vi "Set US Genomics.vi"(8 "error in (no error)":errorcluster, 10 "height":i32, 11 "width":i32) -> (0 "error out":errorcluster, 3 "function return":u32)   [LabVIEW 2014, in "atmcd32d.lvlib"]
doc: "unsigned int WINAPI SetUSGenomics(long width, long height);"
uses:
  atmcd32d.lvlib
  atmcd32d.dll
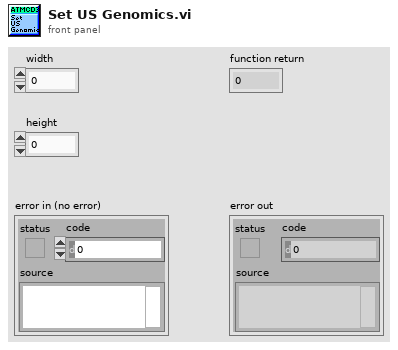
[diagram p1: front panel]
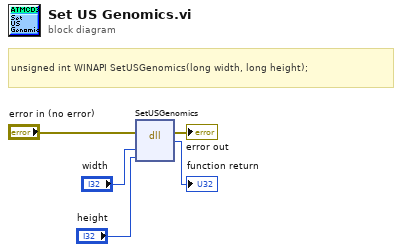
[diagram p0: block diagram]
diagram:
  # "unsigned int WINAPI SetUSGenomics(long width, long height);"
  n1 = dll-call lib="C:/Users/Bakir/Documents/Lambda2-Testing/lib/Andorlib/atmcd32d.*" fn="SetUSGenomics"(error in="error in (no error)", "width"="width", "height"="height") -> (error out=→"error out":errorcluster, →"function return":u32)  [unwired: 4 in, 1 out]
